vi "1-12.vi"(1 "数值 2":dbl) -> (0 "数值":dbl)   [LabVIEW 2022 SP3]
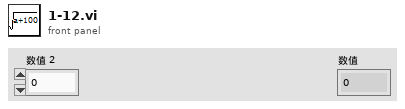
[diagram p1: front panel]
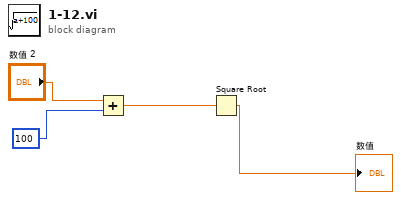
[diagram p0: block diagram]
diagram:
  n1 = Add(x="数值 2", y=100) -> (x+y=w3:dbl)
  n2 = Square Root(x=w3) -> (sqrt(x)=→"数值":dbl)
